vi "niFPGA_U32 Divide (U8).vi"(2 "D [U32.n]":u32, 3 "N [U32.n]":u32) -> (1 "N/D [U8.0]":u8 format="%.0x")   [LabVIEW 2017]
uses:
  <vilib>/Platform/TimedLoop/XDataNode/timing_clust.ctl
  <vilib>/Platform/TimedLoop/XDataNode/nitl_modes.ctl
  <vilib>/Platform/TimedLoop/XDataNode/wakeup.ctl
  <vilib>/Platform/TimedLoop/XDataNode/XDataNode.xnode
  <vilib>/Platform/TimedLoop/XDataNode/XDNodeRunTimeDep.lvlib
panel:
  # "N <= D"
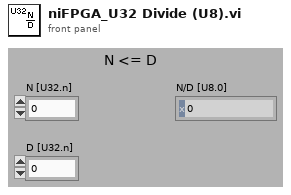
[diagram p1: front panel]
types:
  T1 = typedef "XDNodeRunTimeDep.lvlib/timing_clust.ctl" = cluster{"Expected End [f-1]":u64, "Actual End [f-1]":u64, "Finished Late? [f-1]":bool, "Expected End [i-1]":u64, "Actual End [i-1]":u64, "Finished Late? [i-1]":bool, "Expected Start [i]":u64, "Actual Start [i]":u64, "Expected Start [f]":u64, "Actual Start [f]":u64, "Source Name":string, "Structure Name":string, "Period":i64, "Deadline":i64, "Offset":i64, "Start":i64, "Priority":i32, "Timeout":i32, "Mode":T2, "Wakeup Reason":T3, "Error":errorcluster, "Source Type":string, "Secondary Source Type":string, "Global End Time":u64, "Global Start Time":u64, "Frame Duration":u64, "Iteration Duration":u64, "Assigned CPU":i32, "I/O Scan Engine Mode":u32}
  T2 = typedef "XDNodeRunTimeDep.lvlib/nitl_modes.ctl" = enum32{"No Change", "Process missed periods, maintain original phase", "Discard missed periods, maintain original phase", "Process missed periods, ignore original phase", "Discard missed periods, ignore original phase"}
  T3 = typedef "XDNodeRunTimeDep.lvlib/wakeup.ctl" = enum32{"Normal", "Aborted", "Asynchronous wakeup", "Timing source error", "Timed loop error", "Timeout"}
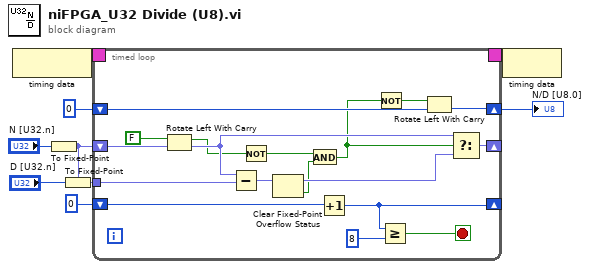
[diagram p0: block diagram]
diagram:
  n1 = node-c288() -> (w9:T1)
  n2 = To Fixed-Point(number="N [U32.n]") -> (fixed-point=w1:fxp<+,32,32>)  [unwired: 1 out]
  n3 = To Fixed-Point(fixed-point type=w1, number="D [U32.n]") -> (fixed-point=w2:fxp<+,32,32>)
  n4 = timed-loop {
    shift-right: [w21] -> _
    shift-left: w1 -> [w23]
    tunnel: w2 -> [w22]
    shift-right: [w26] -> _
    shift-left: u8 0 -> [w27]
    timing: w9 -> [_]
    timing-out: [_] -> w8
    shift-right: [w20] -> w6
    shift-left: u8 0 -> [w16]
    stop <- w24 stop-if-true
    n5 = Rotate Left With Carry(2:w23, 3:FALSE ("carry")) -> (0:w18:fxp<+,32,32>, 1:w14:bool)
    n6 = Subtract(x=w18, y=w22) -> (x-y=w19:fxp<+,32,32>)
    n7 = Not(x=w14) -> (.not. x?=w13:bool)
    n8 = Clear Fixed-Point Overflow Status(3:w19) -> (0:w10:bool, 1:w11:fxp<+,32,32>)
    n9 = And(x=w13, y=w10) -> (x .and. y?=w12:bool)
    n10 = Increment(x=w27) -> (x+1=w26:u8)
    n11 = Not(x=w12) -> (.not. x?=w17:bool)
    n12 = Greater Or Equal?(x=w26, y=u8 8) -> (x >= y?=w24:bool)
    n13 = Rotate Left With Carry(2:w16, 3:w17) -> (0:w20:u8)  [unwired: 1 out]
    n14 = Select(t=w18, s=w12, f=w11) -> (s? t:f=w21:fxp<+,32,32>)
  }
  "N/D [U8.0]" <- w6
  n15 = node-c288(w8) -> ()
